vi "p10.vi"() -> ()   [LabVIEW 2015]
panel:
  out "Appended String":string
  out "Array[Index] String":string
  out "offset past match":i32
  out "Replaced string":string
  out "token index":i32
  out "token string":string
  out "offset past token":i32
  out "string out":string
  out "selection":bool
  out "Match String":string
  out "length":i32
  out "index":i32
  out "Match First String":string
  out "Picked Line":string
  out "offset of match":i32
  out "match + rest of string":string
  out "substring before match":string
  out "value":dbl
  out "Remaining string":string
  out "Converted Number":u32
  out "offset past number":i32
  out "output string":string
  out "Engineering string":string
  out "E-format string":string
  out "F-format string":string
  out "F-format string":string
  out "octal integer string":string
  out "octal integer string":string
  out "hex integer string":string
  out "hex integer string":string
  out "decimal integer string":string
  out "decimal integer string":string
  # "MATCH T/F STRING"
  # "NUMBER TO STRING"
  # "SEARCH/SPLIT STRING"
  # "SCAN STRING FOR TOKENS"
  # "STRING TO NUMBER"
  # "SEARCH & REPLACE STRING"
  # "PICK A LINE"
  # "NUMBER TO STRING"
  # "NUMBER TO STRING"
  # "INDEX STRING ARRAY"
  # "APPEND T/F STRING"
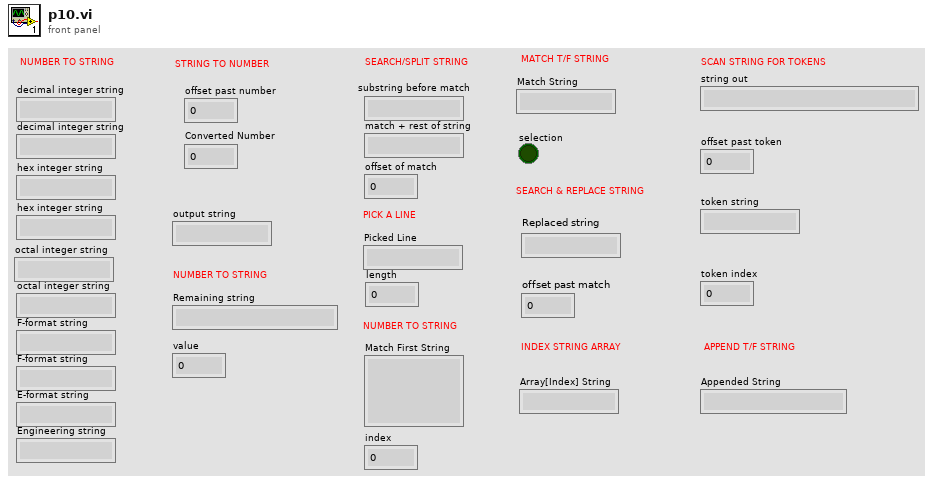
[diagram p1: front panel]
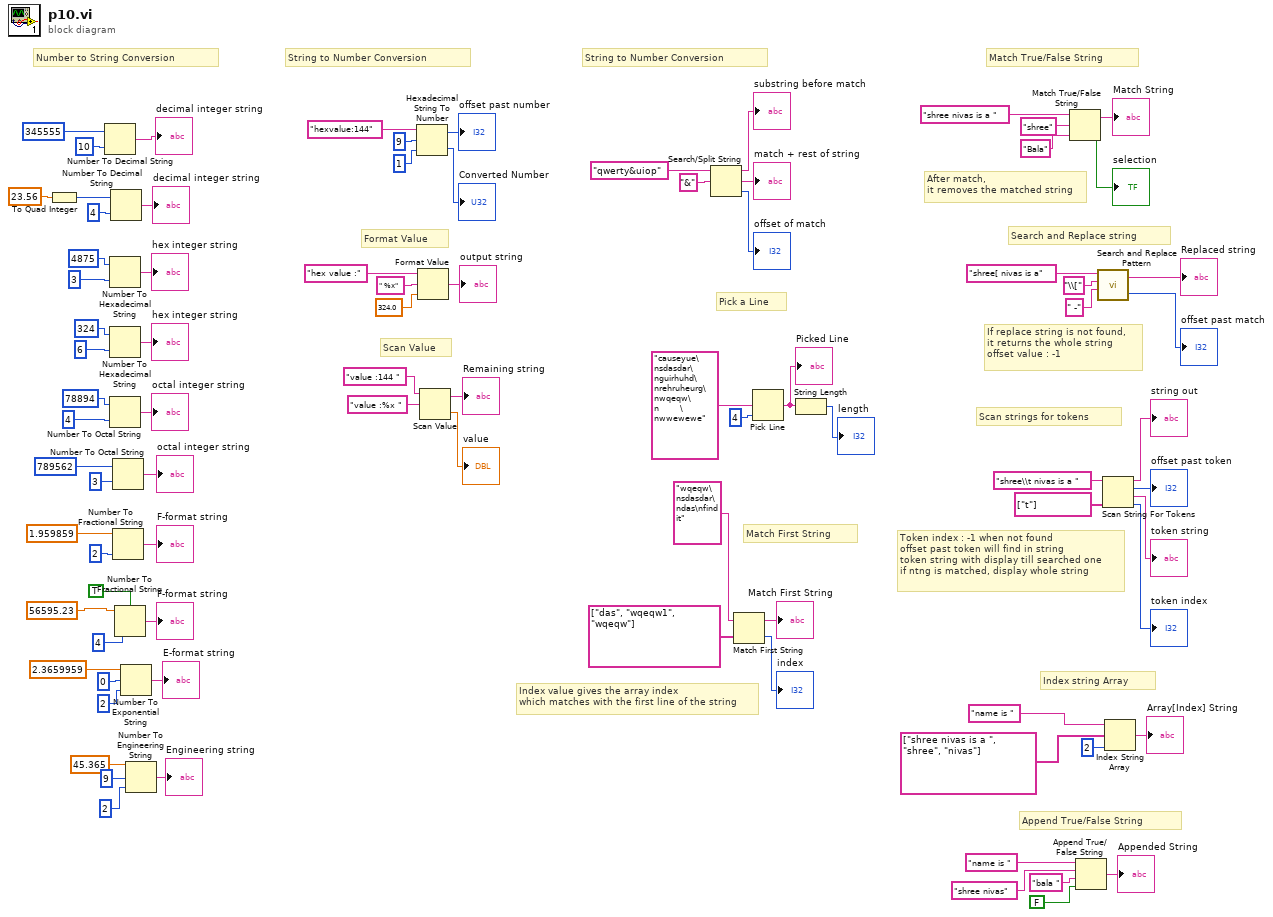
[diagram p0: block diagram]
diagram:
  w39 = 4 ("number")
  # "Token index : -1 when not found\noffset past token will find in string\ntoken string with display till searched one\nif ntng is matched, display whole string"
  # "If replace string is not found, \nit returns the whole string \noffset value : -1"
  # "After match, \nit removes the matched string"
  # "Append True/False String"
  # "Index string Array"
  # "Search and Replace string"
  # "Scan strings for tokens"
  # "Match True/False String"
  # "Index value gives the array index\nwhich matches with the first line of the string"
  # "Match First String"
  # "Pick a Line"
  # "String to Number Conversion"
  # "Scan Value"
  # "Format Value"
  # "String to Number Conversion"
  # "Number to String Conversion"
  n1 = To Quad Integer(1:23.56 ("number")) -> (0:w79:i64)
  n2 = Number To Decimal String(number=345555, width (-)=10 ("number")) -> (decimal integer string=→"decimal integer string":string)
  n3 = Number To Hexadecimal String(1:3 ("number"), 2:4875 ("number")) -> (0:→"hex integer string":string)
  n4 = Number To Hexadecimal String(1:6 ("number"), 2:324 ("number")) -> (0:→"hex integer string":string)
  n5 = Number To Octal String(1:4 ("number"), 2:78894 ("number")) -> (0:→"octal integer string":string)
  n6 = Number To Decimal String(number=w79, width (-)=4 ("number")) -> (decimal integer string=→"decimal integer string":string)
  n7 = Number To Octal String(1:3 ("number"), 2:789562 ("number")) -> (0:→"octal integer string":string)
  n8 = Number To Fractional String(number=1.959859, precision (6)=2 ("number")) -> (F-format string=→"F-format string":string)  [unwired: 2 in]
  n9 = Number To Fractional String(use system decimal point (T)=TRUE, number=56595.23, width (-)=w39, precision (6)=w39) -> (F-format string=→"F-format string":string)
  n10 = Number To Exponential String(number=2.3659959, precision (6)=2 ("number"), 3:0 ("number")) -> (E-format string=→"E-format string":string)  [unwired: 1 in]
  n11 = Number To Engineering String(2:2 ("number"), 3:9 ("number"), 4:45.365 ("number")) -> (0:→"Engineering string":string)  [unwired: 1 in]
  n12 = Hexadecimal String To Number(string="hexvalue:144" ("string (\"\")"), offset=9, default (0uL)=u32 1 ("default (0 U32)")) -> (offset past number=→"offset past number":i32, number=→"Converted Number":u32)
  n13 = Format Value(string ("")="hex value :", format string=" %x", value (0)=324.0) -> (output string=→"output string":string)
  n14 = Scan Value(string="value :144 ", format string="value :%x ") -> (output string=→"Remaining string":string, value=→"value":dbl)  [unwired: 1 in]
  n15 = Search/Split String(string="qwerty&uiop", search string/char (-)="&") -> (substring before match=→"substring before match":string, match + rest of string=→"match + rest of string":string, offset of match=→"offset of match":i32)  [unwired: 1 in]
  n16 = Match First String(2:string[] ["das", "wqeqw1", "wqeqw"] ("string array"), 3:"wqeqw\nsdasdar\ndas\nfind it" ("multi-line string")) -> (0:→"index":i32, 1:→"Match First String":string)
  n17 = Pick Line(multi-line string="causeyue\nsdasdar\nguirhuhd\nrehruheurg\nwqeqw\n       \nwwewewe", line index=4) -> (output string=w27:string)  [unwired: 1 in]
  "Picked Line" <- w27
  n18 = String Length(string=w27) -> (length=→"length":i32)
  n19 = Match True/False String(2:"Bala" ("string"), 3:"shree" ("string"), 4:"shree nivas is a " ("string")) -> (0:→"selection":bool, 1:→"Match String":string)
  n20 = Append True/False String(1:FALSE ("selector"), 2:"bala " ("string (\"\")"), 3:"shree nivas" ("string (\"\")"), 4:"name is " ("string (\"\")")) -> (0:→"Appended String":string)
  n21 = call <vilib>:"Search and Replace Pattern.vi"("string"="shree[ nivas is a", "regular expression (\"\")"="\\[" ("regular expression (\"\")"), "replace string (\"\")"=" -" ("replace string (\"\")")) -> ("result string"=→"Replaced string":string, "offset past match"=→"offset past match":i32)  [unwired: 2 in]
  n22 = Scan String For Tokens(6:string[] ["t"] ("delimiters (\\s,\\t,\\r,\\n)"), 9:"shree\\t nivas is a " ("string")) -> (0:→"token index":i32, 1:→"token string":string, 2:→"offset past token":i32, 3:→"string out":string)  [unwired: 4 in]
  n23 = Index String Array(1:2 ("index"), 2:string[] ["shree nivas is a ", "shree", "nivas"] ("delimiters (\\s,\\t,\\r,\\n)"), 3:"name is " ("string (\"\")")) -> (0:→"Array[Index] String":string)
